vi "Inverse f Correct MagdB for Exponent and Gain.vi"(6 "alignment frequency (Hz)":dbl format="%.2g", 9 "exponent":dbl=1.0 format="%.2g", 10 "unity gain freq (rd/s)":dbl=1.0 format="%.2g", 11 "magnitude (dB)":T1) -> (1 "gain to apply":dbl=1.0 format="%.2g", 2 "corrected magnitude (dB)":T1, 3 "magnitude error (dB)":T1)   [LabVIEW 2014, in "NI_AALBase.lvlib"]
uses:
  NI_AALBase.lvlib
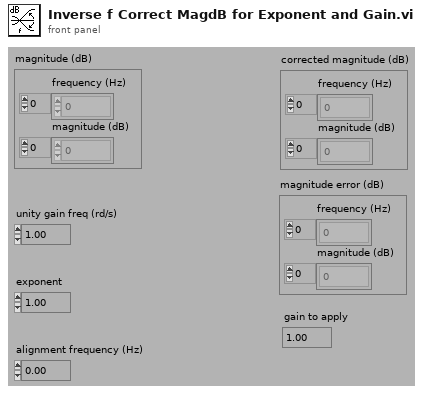
[diagram p1: front panel]
types:
  T1 = cluster{"frequency (Hz)":dbl[], "magnitude (dB)":dbl[]}
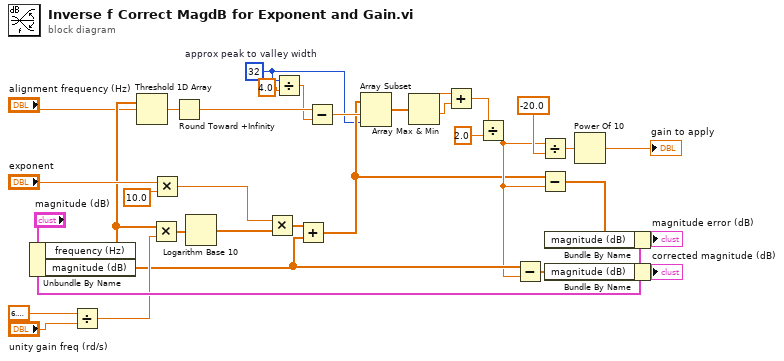
[diagram p0: block diagram]
diagram:
  w1 = 32  # approx peak to valley width
  n1 = Unbundle By Name("magnitude (dB)") -> ("frequency (Hz)"=w16:dbl[], "magnitude (dB)"=w13:dbl[])
  n2 = Divide(x=6.283185307179586, y="unity gain freq (rd/s)") -> (x/y=w23:dbl)
  n3 = Threshold 1D Array(2:"alignment frequency (Hz)", 3:w16) -> (0:w15:dbl)  [unwired: 1 in]
  n4 = Multiply(x=w16, y=w23) -> (x*y=w17:dbl[])
  n5 = Multiply(x="exponent", y=10.0) -> (x*y=w31:dbl)
  n6 = Round Toward +Infinity(x=w15) -> (ceil(x): smallest int >= x=w11:dbl)
  n7 = Logarithm Base 10(1:w17) -> (0:w20:dbl[])
  n8 = Multiply(x=w31, y=w20) -> (x*y=w30:dbl[])
  n9 = Divide(x=w1, y=4.0) -> (x/y=w2:dbl)
  n10 = Add(x=w30, y=w13) -> (x+y=w4:dbl[])
  n11 = Subtract(x=w11, y=w2) -> (x-y=w12:dbl)
  n12 = Array Subset(array=w4, index=w12, length=w1) -> (w10:dbl[])
  n13 = Array Max & Min(array=w10) -> (max value=w9:dbl, min value=w8:dbl)  [unwired: 2 out]
  n14 = Add(x=w9, y=w8) -> (x+y=w6:dbl)
  n15 = Divide(x=w6, y=2.0) -> (x/y=w5:dbl)
  n16 = Subtract(x=w13, y=w5) -> (x-y=w19:dbl[])
  n17 = Divide(x=w5, y=-20.0) -> (x/y=w26:dbl)
  n18 = Subtract(x=w4, y=w5) -> (x-y=w28:dbl[])
  n19 = Bundle By Name(cluster="magnitude (dB)", "magnitude (dB)"=w28) -> (→"magnitude error (dB)":T1)
  n20 = Bundle By Name(cluster="magnitude (dB)", "magnitude (dB)"=w19) -> (→"corrected magnitude (dB)":T1)
  n21 = Power Of 10(x=w26) -> (10^x=→"gain to apply":dbl)
